vi "create.vi"(11 "result":refnum<class "result.lvclass">) -> (3 "actor message report":refnum<class "actor message report.lvclass">)   [LabVIEW 2014, in "actor message report.lvclass"]
uses:
  actor message report.lvclass
  result/result.lvclass
  actor message report.lvclass/actor message report.ctl
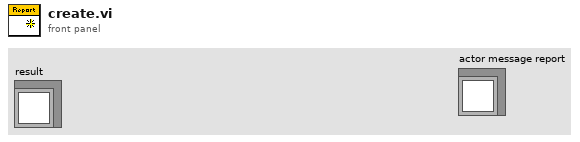
[diagram p1: front panel]
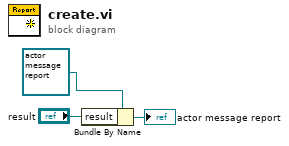
[diagram p0: block diagram]
diagram:
  n1 = Bundle By Name(cluster=refnum<class "actor message report.lvclass"> refnum ("actor message report in"), "result"="result") -> (→"actor message report":refnum<class "actor message report.lvclass">)
